vi "Autonomous Independent.vi"   [LabVIEW 2014]
doc: "This VI is called when autonomous begins, and will automatically be terminated when autonomous ends. You can carry out timed or sensor driven robot movement independently without needing to return to the caller."
uses:
  1756_Code/General_VI/Global Var.vi
panel:
  # "Be sure to right-click and choose Data Operations>>Make Current Value default if you want to save the array values with the VI"
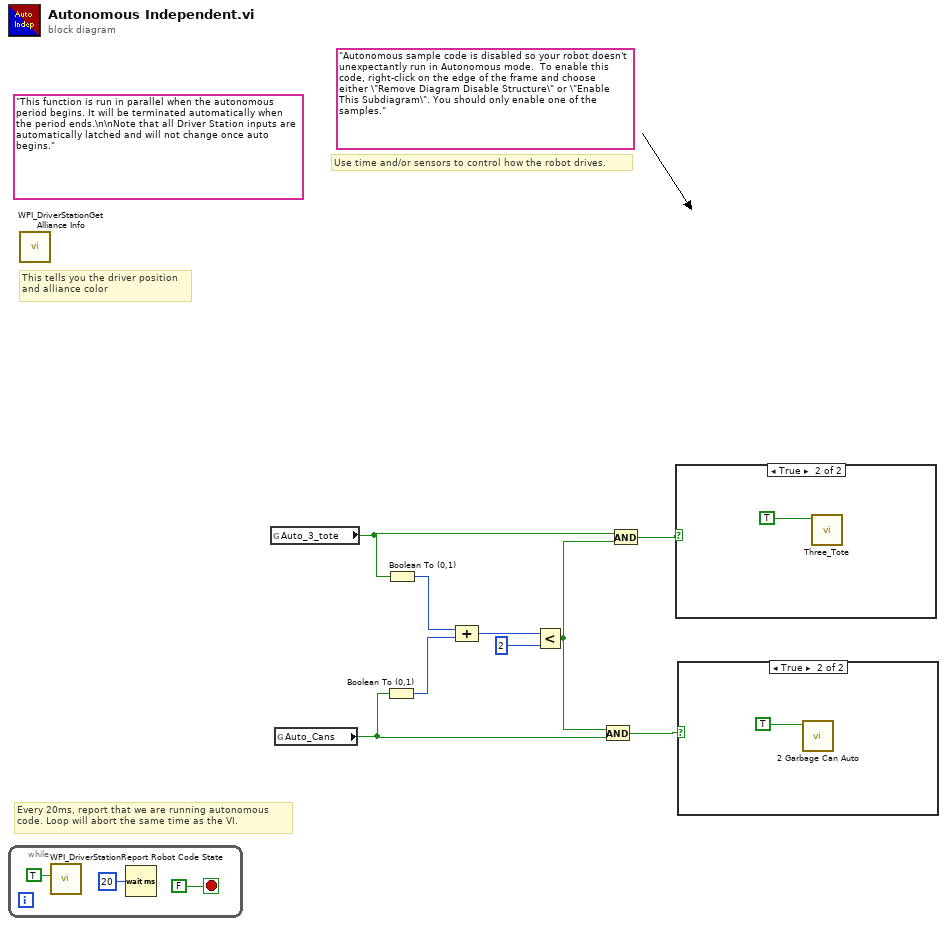
[diagram p0: block diagram]
diagram:
  (unwired) "Autonomous sample code is disabled so your robot doesn't unexpectantly run in Autonomous mode.  To enable this code, right-click on the edge of the frame and choose either \"Remove Diagram Disable Structure\" or \"Enable This Subdiagram\". You should only enable one of the samples."
  (unwired) "This function is run in parallel when the autonomous period begins. It will be terminated automatically when the period ends.\n\nNote that all Driver Station inputs are automatically latched and will not change once auto begins."
  # "Every 20ms, report that we are running autonomous\ncode. Loop will abort the same time as the VI."
  # "Use time and/or sensors to control how the robot drives."
  # "This tells you the driver position\nand alliance color"
  n1 = while {
    stop <- FALSE stop-if-true
    n2 = call <vilib>:"WPI_DriverStationReport Robot Code State.vi"("Autonomous"=TRUE) -> ()  [unwired: 10 in, 1 out]
    n3 = Wait (ms)(milliseconds to wait=u32 20) -> ()  [unwired: 1 out]
  }
  n4 = call <vilib>:"WPI_DriverStationGet Alliance Info.vi"() -> ()  [unwired: 12 out]
  n5 = global read "Global Var.vi" "Auto_3_tote"() -> (w2:bool)
  n6 = global read "Global Var.vi" "Auto_Cans"() -> (w3:bool)
  n7 = Boolean To (0,1)(Boolean=w3) -> (0, 1=w7:i16)
  n8 = Boolean To (0,1)(Boolean=w2) -> (0, 1=w8:i16)
  n9 = Compound Arithmetic op=ADD(w8, w7) -> (w6:i16)
  n10 = Less?(x=w6, y=i16 2) -> (x < y?=w1:bool)
  n11 = And(x=w1, y=w3) -> (x .and. y?=w4:bool)
  n12 = And(x=w2, y=w1) -> (x .and. y?=w5:bool)
  n13 = case shown="True" w5 {
    frame False {
    }
    frame True {
      n14 = call "Three_Tote.vi"("3_Tote_Enable"=TRUE) -> ()  [unwired: 11 in]
    }
  }
  n15 = case shown="True" w4 {
    frame False {
    }
    frame True {
      n16 = call "2 Garbage Can Auto.vi"("Can Auto Enable"=TRUE ("3_Tote_Enable")) -> ()  [unwired: 11 in]
    }
  }
